vi "merlin.vi"() -> ()   [LabVIEW 2018]
uses:
  classes/Tushars Events Toolkit/Software/Modules/EventClient_ObjectReference.ctl
  Strict Type Controls/Settings Operation.ctl
  <vilib>/Instr/_visa.llb/VISA Configure Serial Port (Instr).vi
  classes/Variable Manager/VariableManager_Bool.vi
  classes/Variable Manager/VariableManager_Double.vi
panel:
  out "Quit":bool
  out "error out":errorcluster
  in  "error in (no error)":errorcluster
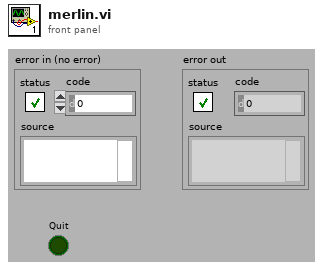
[diagram p1: front panel]
types:
  T1 = typedef "EventClient_ObjectReference.ctl" = refnum<k1>
  T2 = typedef "Settings Operation.ctl" = enum8{"Get Value", "Set Value", "Read File", "Write File", "Write Stored Value"}
  T3 = cluster{"#Stages":enum16{"None", "1 Pole", "2 Pole"}, "Phase":enum16{"1 Phase", "2 Phase"}, "SyncMode":enum16{"Int Chop Off", "Int Chop On", "Ext Chop Off", "Ext Chop On"}, "Time Const":enum16{".003s", ".010s", ".030s", ".100s", ".300s", "1.00s", "3.00s", "10.0s", "30.0s", "100s"}}
  T4 = enum16{"Int Chop Off", "Int Chop On", "Ext Chop Off", "Ext Chop On"}
  T5 = enum16{".003s", ".010s", ".030s", ".100s", ".300s", "1.00s", "3.00s", "10.0s", "30.0s", "100s"}
  T6 = typedef "Settings.ctl" = cluster{"Mono Cr":cluster{"Port":refnum<visa-resource-name>, "baud rate":u32, "data bits":u16, "parity":enum16{"None", "Odd", "Even", "Mark", "Space"}, "stop bits":u16, "flow control":u16, "timeout":u32}, "Merlin":cluster{"Port":refnum<visa-resource-name>, "baud rate":u32, "data bits":u16, "parity":enum16{"None", "Odd", "Even", "Mark", "Space"}, "stop bits":u16, "flow control":u16, "timeout":u32}}
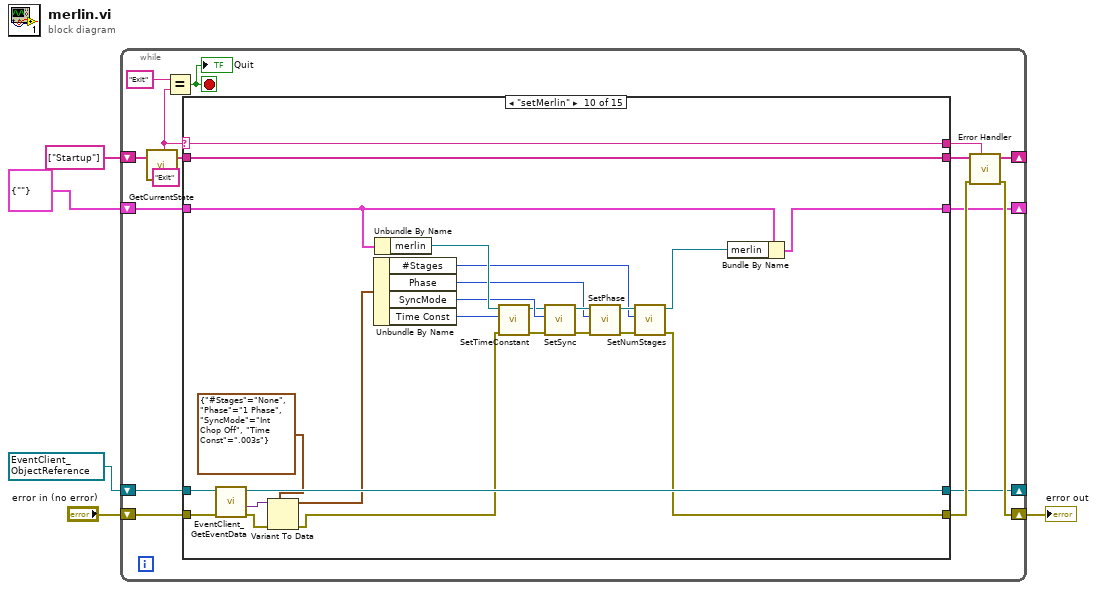
[diagram p0: block diagram]
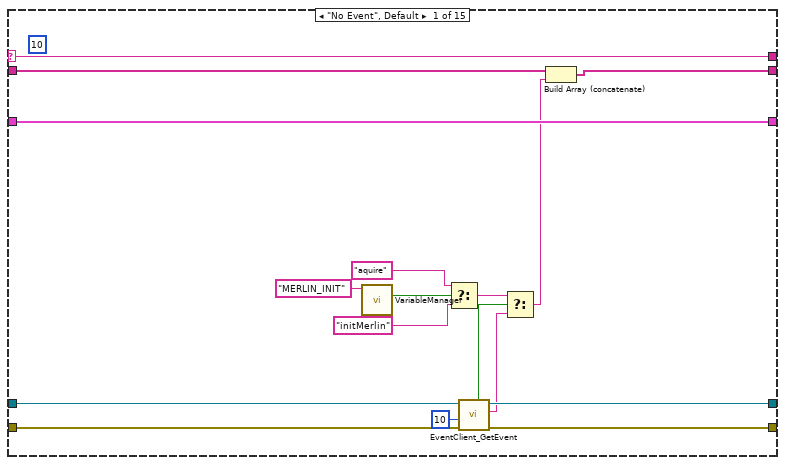
[diagram p2: hidden frame]
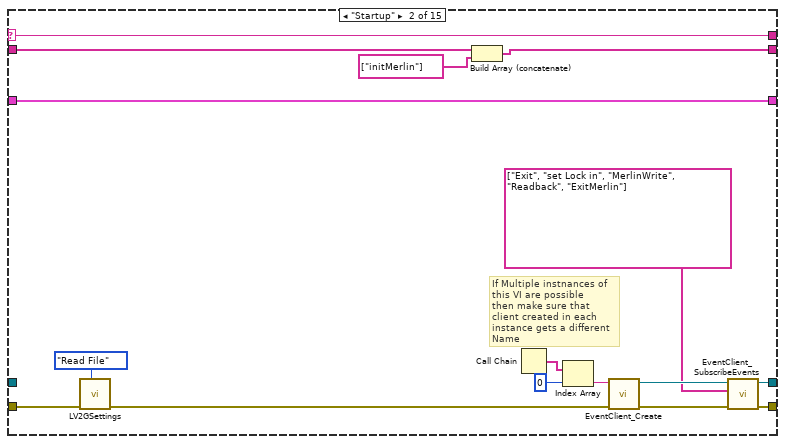
[diagram p3: hidden frame]
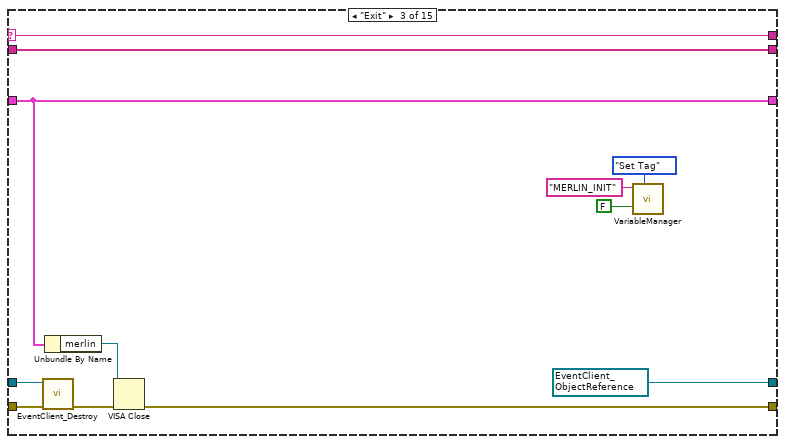
[diagram p4: hidden frame]
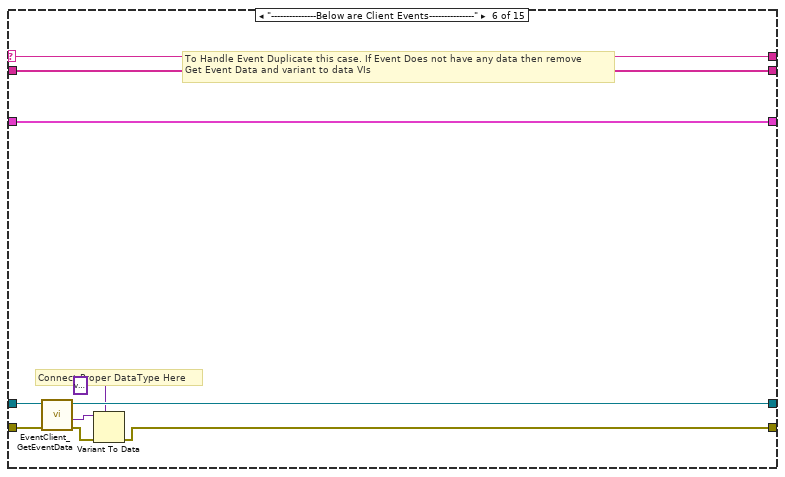
[diagram p7: hidden frame]
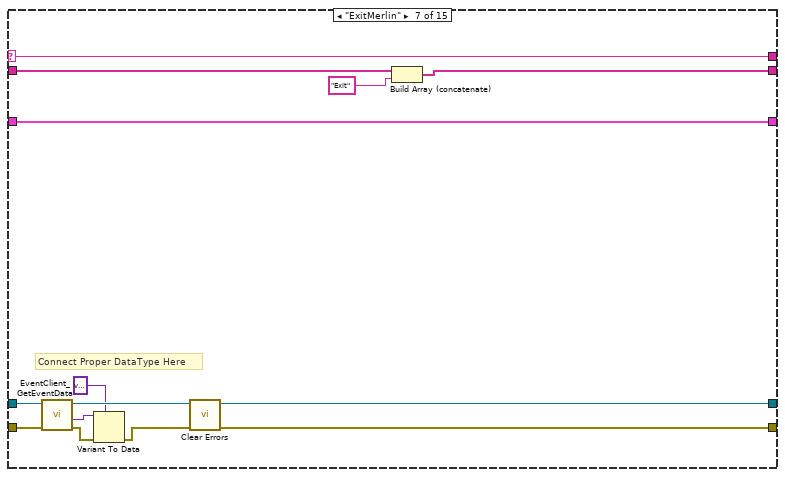
[diagram p8: hidden frame]
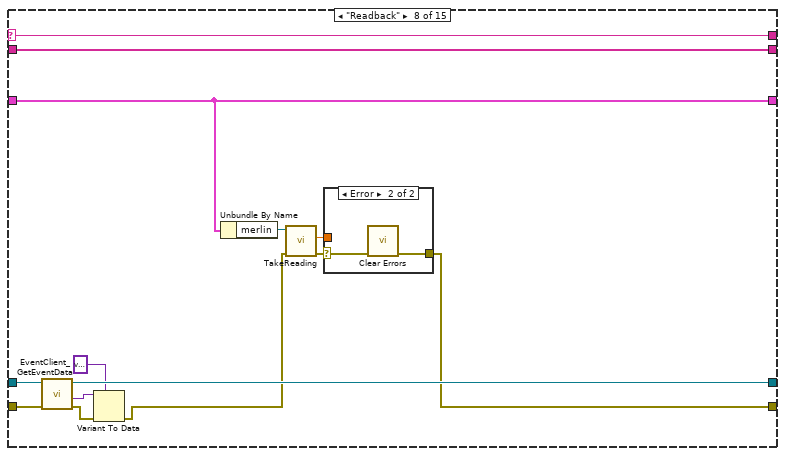
[diagram p9: hidden frame]
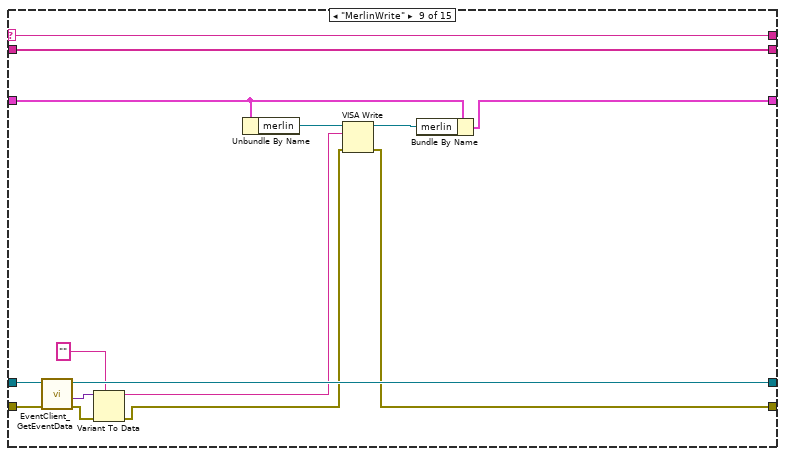
[diagram p11: hidden frame]
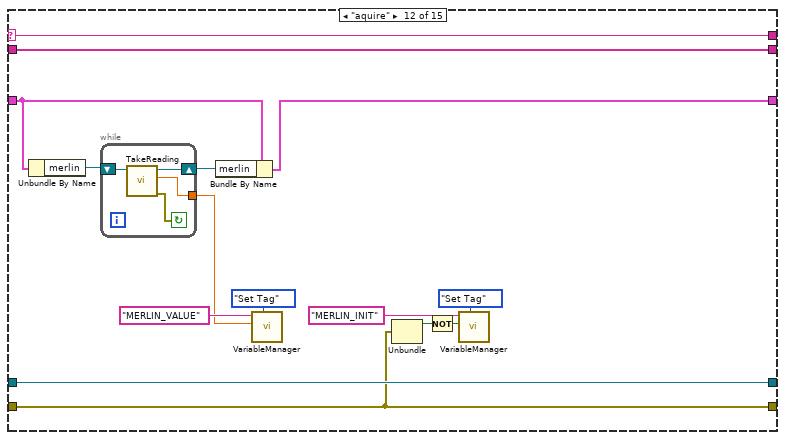
[diagram p13: hidden frame]
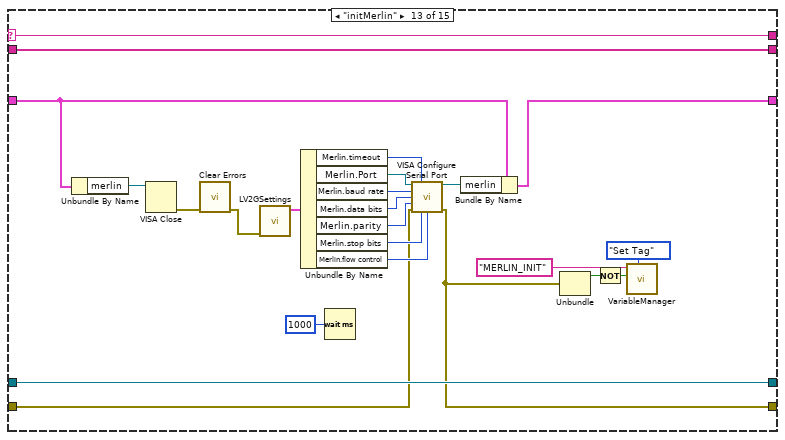
[diagram p14: hidden frame]
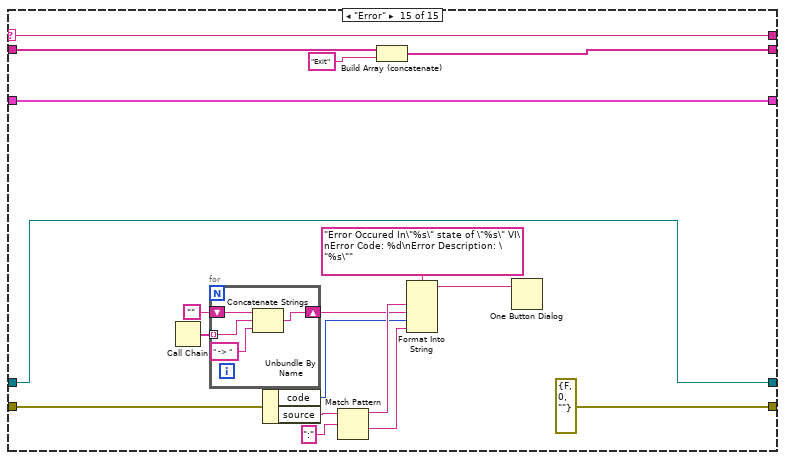
[diagram p16: hidden frame]
diagram:
  w2 = T1 refnum items=["EventClient"] ("reference")
  n1 = while {
    shift-right: [w16] -> _
    shift-left: string[] ["Startup"] ("State Array Out") -> [w20]
    shift-right: [w12] -> w3
    shift-left: "error in (no error)" -> [w13]
    shift-right: [w9] -> _
    shift-left: w2 -> [w8]
    shift-right: [w6] -> _
    shift-left: cluster{"merlin":refnum<visa-resource-name>} {"merlin"=""} -> [w7]
    stop <- w17 stop-if-true
    (unwired) "Exit" ("x")
    n2 = call "GetCurrentState.vi"("State Array In"=w20) -> ("Current State"=w10:string, "State Array Out"=w19:string[])  [unwired: 17 in]
    n3 = Equal?(x="Exit", y=w10) -> (x = y?=w17:bool)
    "Quit" <- w17
    n4 = case shown="\"setMerlin\"" w10 {
      selector: w10 -> [w37 w53 w65 w69 w74 w84 w97 w111 w129 w154 w159 w174 w202 w208 w226]
      tunnel: w19 -> [w29 w52 w64 w70 w75 w85 w98 w112 w130 w155 w160 w175 w203 w207 w213]
      tunnel: [w32 w51 w64 w70 w75 w85 w88 w112 w130 w155 w160 w175 w203 w207 w210] -> w15
      tunnel: [w34 w45 w59 w68 w73 w80 w86 w99 w116 w133 w158 w169 w182 w206 errorcluster {"status"=FALSE, "code"=0, "source"=""} ("error in (no error)")] -> w11
      tunnel: [w37 w53 w65 w69 w74 w84 w97 w111 w129 w154 w159 w174 w202 w208 w226] -> w14
      tunnel: w13 -> [w35 w40 w62 w68 w73 w82 w95 w109 w127 w152 w158 w169 w186 w206 w214]
      tunnel: [w33 w43 w61 w67 w72 w78 w91 w106 w124 w149 w157 w173 w201 w205 w212] -> w9
      tunnel: w8 -> [w36 _ w63 w67 w72 w83 w96 w110 w128 w153 w157 w173 w201 w205 w212]
      tunnel: w7 -> [w30 w41 w58 w66 w71 w76 w89 w101 w121 w145 w156 w166 w189 w204 w211]
      tunnel: [w30 w41 w58 w66 w71 w76 w89 w101 w122 w146 w156 w165 w188 w204 w211] -> w6
      frame "No Event", Default {
        (unwired) 10
        n5 = call-poly "VariableManager.vi"("Tag"="MERLIN_INIT") -> ("Value out"=w27:bool)  [unwired: 7 in, 3 out]
        n6 = Select(t="aquire" ("Tag"), s=w27, f="initMerlin" ("Tag")) -> (s? t:f=w23:string)
        n7 = call "EventClient_GetEvent.vi"("error in (no error)"=w35, "timeout in ms (-1)"=10, "reference"=w36) -> ("error out"=w34:errorcluster, "Name"=w22:string, "reference out"=w33:T1, "timed out?"=w24:bool)  [unwired: 4 in, 1 out]
        n8 = Select(t=w23, s=w24, f=w22) -> (s? t:f=w21:string)
        n9 = Build Array (concatenate)(w29, w21) -> (w32:string[])
      }
      frame "Startup" {
        # "If Multiple instnances of this VI are possible \nthen make sure that client created in each instance gets a different Name"
        n10 = call "LV2GSettings.vi"("Operation"=Settings_Operation."Read File", "error in (no error)"=w40) -> ("error out"=w39:errorcluster)  [unwired: 8 in, 1 out]
        n11 = Build Array (concatenate)(w52, string[] ["initMerlin"] ("State Array Out")) -> (w51:string[])
        n12 = Call Chain() -> (call chain=w49:string[])
        n13 = Index Array(array=w49, index=0) -> (element=w47:string)
        n14 = call "EventClient_Create.vi"("error in (no error)"=w39, "Instance Name"=w47) -> ("error out"=w46:errorcluster, "reference"=w44:T1)  [unwired: 8 in]
        n15 = call "EventClient_SubscribeEvents.vi"("error in (no error)"=w46, "Events"=string[] ["Exit", "set Lock in", "MerlinWrite", "Readback", "ExitMerlin"], "reference"=w44) -> ("error out"=w45:errorcluster, "reference out"=w43:T1)  [unwired: 7 in]
      }
      frame "Exit" {
        w61 = T1 refnum items=["EventClient"] ("reference out")
        n16 = call "EventClient_Destroy.vi"("error in (no error)"=w62, "reference"=w63) -> ("error out"=w60:errorcluster)  [unwired: 9 in]
        n17 = Unbundle By Name(w58) -> ("merlin"=w57:refnum<visa-resource-name>)
        n18 = VISA Close(VISA resource name=w57, error in (no error)=w60) -> (error out=w59:errorcluster)
        n19 = call-poly "VariableManager.vi"("Operation"=enum16{"Get Tag", "Set Tag"}."Set Tag", "Value"=FALSE, "Tag"="MERLIN_INIT") -> ()  [unwired: 5 in, 4 out]
      }
      frame "---------------Below are UI Events---------------" {
        # "This State will never Execute\nIt is added just for improving code readability please do not remove this case"
      }
      frame "---------------Below are Menu Events---------------" {
        # "This State will never Execute\nIt is added just for improving code readability please do not remove this case"
      }
      frame "---------------Below are Client Events---------------" {
        # "To Handle Event Duplicate this case. If Event Does not have any data then remove\nGet Event Data and variant to data VIs"
        # "Connect Proper DataType Here"
        n20 = call "EventClient_GetEventData.vi"("error in (no error)"=w82, "reference"=w83) -> ("error out"=w81:errorcluster, "Data"=w79:variant, "reference out"=w78:T1)  [unwired: 7 in]
        n21 = Variant To Data(error in=w81, type=variant, Variant=w79) -> (error out=w80:errorcluster)  [unwired: 1 out]
      }
      frame "ExitMerlin" {
        # "Connect Proper DataType Here"
        n22 = call "EventClient_GetEventData.vi"("error in (no error)"=w95, "reference"=w96) -> ("error out"=w94:errorcluster, "Data"=w92:variant, "reference out"=w91:T1)  [unwired: 7 in]
        n23 = Variant To Data(error in=w94, type=variant, Variant=w92) -> (error out=w93:errorcluster)  [unwired: 1 out]
        n24 = call <vilib>:"Clear Errors.vi"("error in (no error)"=w93) -> ("error out"=w86:errorcluster)  [unwired: 5 in, 1 out]
        n25 = Build Array (concatenate)(w98, "Exit" ("x")) -> (w88:string[])
      }
      frame "Readback" {
        n26 = call "EventClient_GetEventData.vi"("error in (no error)"=w109, "reference"=w110) -> ("error out"=w108:errorcluster, "Data"=w107:variant, "reference out"=w106:T1)  [unwired: 7 in]
        n27 = Variant To Data(error in=w108, type=variant, Variant=w107) -> (error out=w100:errorcluster)  [unwired: 1 out]
        n28 = Unbundle By Name(w101) -> ("merlin"=w104:refnum<visa-resource-name>)
        n29 = call "TakeReading.vi"("error in"=w100, "Port"=w104) -> ("error out"=w103:errorcluster, "Voltage(mV)"=w102:dbl)  [unwired: 6 in, 2 out]
        n30 = case shown="Error" w103 {
          selector: w103 -> [w113 w115]
          tunnel: w102 -> [_ _]
          tunnel: [w113 w114] -> w99
          frame No Error {
          }
          frame Error {
            n31 = call <vilib>:"Clear Errors.vi"("error in (no error)"=w115) -> ("error out"=w114:errorcluster)  [unwired: 5 in, 1 out]
          }
        }
      }
      frame "MerlinWrite" {
        n32 = call "EventClient_GetEventData.vi"("error in (no error)"=w127, "reference"=w128) -> ("error out"=w126:errorcluster, "Data"=w125:variant, "reference out"=w124:T1)  [unwired: 7 in]
        n33 = Variant To Data(error in=w126, type="", Variant=w125) -> (data=w118:string, error out=w117:errorcluster)
        n34 = Unbundle By Name(w121) -> ("merlin"=w120:refnum<visa-resource-name>)
        n35 = VISA Write(VISA resource name=w120, write buffer=w118, error in (no error)=w117) -> (VISA resource name out=w119:refnum<visa-resource-name>, error out=w116:errorcluster)  [unwired: 1 out]
        n36 = Bundle By Name(cluster=w121, "merlin"=w119) -> (w122:cluster{"merlin":refnum<visa-resource-name>})
      }
      frame "setMerlin" {
        n37 = call "EventClient_GetEventData.vi"("error in (no error)"=w152, "reference"=w153) -> ("error out"=w151:errorcluster, "Data"=w150:variant, "reference out"=w149:T1)  [unwired: 7 in]
        n38 = Variant To Data(error in=w151, type=T3 {"#Stages"=enum."None", "Phase"=enum."1 Phase", "SyncMode"=enum."Int Chop Off", "Time Const"=enum.".003s"}, Variant=w150) -> (data=w147:T3, error out=w134:errorcluster)
        n39 = Unbundle By Name(w147) -> ("#Stages"=w131:enum16{"None", "1 Pole", "2 Pole"}, "Phase"=w132:enum16{"1 Phase", "2 Phase"}, "SyncMode"=w139:T4, "Time Const"=w141:T5)
        n40 = Unbundle By Name(w145) -> ("merlin"=w140:refnum<visa-resource-name>)
        n41 = call "SetTimeConstant.vi"("error in"=w134, "Time Const"=w141, "Port"=w140) -> ("error out"=w144:errorcluster, "Port out"=w138:refnum<visa-resource-name>)  [unwired: 7 in]
        n42 = call "SetSync.vi"("error in"=w144, "SyncMode"=w139, "Port"=w138) -> ("error out"=w143:errorcluster, "Port out"=w137:refnum<visa-resource-name>)  [unwired: 7 in]
        n43 = call "SetPhase.vi"("error in"=w143, "Phase"=w132, "Port"=w137) -> ("error out"=w142:errorcluster, "Port out"=w136:refnum<visa-resource-name>)  [unwired: 7 in]
        n44 = call "SetNumStages.vi"("error in"=w142, "#Stages"=w131, "Port"=w136) -> ("error out"=w133:errorcluster, "Port out"=w135:refnum<visa-resource-name>)  [unwired: 7 in]
        n45 = Bundle By Name(cluster=w145, "merlin"=w135) -> (w146:cluster{"merlin":refnum<visa-resource-name>})
      }
      frame "---------------Below are Subroutine states---------------" {
      }
      frame "aquire" {
        n46 = Unbundle By Name(w166) -> ("merlin"=w167:refnum<visa-resource-name>)
        n47 = while {
          tunnel: [w177] -> w161
          shift-right: [w176] -> w164
          shift-left: w167 -> [w178]
          stop <- w179 continue-if-true
          n48 = call "TakeReading.vi"("Port"=w178) -> ("error out"=w179:errorcluster, "Voltage(mV)"=w177:dbl, "Port out"=w176:refnum<visa-resource-name>)  [unwired: 7 in, 1 out]
        }
        n49 = Bundle By Name(cluster=w166, "merlin"=w164) -> (w165:cluster{"merlin":refnum<visa-resource-name>})
        n50 = call-poly "VariableManager.vi"("Operation"=enum16{"Get Tag", "Set Tag"}."Set Tag", "Value"=w161, "Tag"="MERLIN_VALUE") -> ()  [unwired: 4 in, 5 out]
        n51 = Unbundle(w169) -> ("status"=w171:bool)  [unwired: 2 out]
        n52 = Not(x=w171) -> (.not. x?=w172:bool)
        n53 = call-poly "VariableManager.vi"("Operation"=enum16{"Get Tag", "Set Tag"}."Set Tag", "Value"=w172, "Tag"="MERLIN_INIT") -> ()  [unwired: 5 in, 4 out]
      }
      frame "initMerlin" {
        n54 = Unbundle By Name(w189) -> ("merlin"=w190:refnum<visa-resource-name>)
        n55 = VISA Close(VISA resource name=w190) -> (error out=w192:errorcluster)  [unwired: 1 in]
        n56 = call <vilib>:"Clear Errors.vi"("error in (no error)"=w192) -> ("error out"=w191:errorcluster)  [unwired: 5 in, 1 out]
        n57 = call "LV2GSettings.vi"("error in (no error)"=w191) -> ("Settings out"=w200:T6)  [unwired: 9 in, 1 out]
        n58 = Unbundle By Name(w200) -> ("Merlin.timeout"=w199:u32, "Merlin.Port"=w193:refnum<visa-resource-name>, "Merlin.baud rate"=w198:u32, "Merlin.data bits"=w197:u16, "Merlin.parity"=w196:enum16{"None", "Odd", "Even", "Mark", "Space"}, "Merlin.stop bits"=w195:u16, "Merlin.flow control"=w194:u16)
        n59 = Wait (ms)(milliseconds to wait=u32 1000) -> ()  [unwired: 1 out]
        n60 = call-poly "VISA Configure Serial Port"("VISA resource name"=w193, "timeout (10sec)"=w199, "baud rate (9600)"=w198, "data bits (8)"=w197, "parity (0:none)"=w196, "error in (no error)"=w186, "stop bits (10: 1 bit)"=w195, "flow control (0:none)"=w194) -> ("VISA resource name out"=w187:refnum<visa-resource-name>, "error out"=w182:errorcluster)  [unwired: 6 in]
        n61 = Bundle By Name(cluster=w189, "merlin"=w187) -> (w188:cluster{"merlin":refnum<visa-resource-name>})
        n62 = Unbundle(w182) -> ("status"=w184:bool)  [unwired: 2 out]
        n63 = Not(x=w184) -> (.not. x?=w185:bool)
        n64 = call-poly "VariableManager.vi"("Operation"=enum16{"Get Tag", "Set Tag"}."Set Tag", "Value"=w185, "Tag"="MERLIN_INIT") -> ()  [unwired: 5 in, 4 out]
      }
      frame "---------------Below are Error Handling VIs---------------" {
      }
      frame "Error" {
        n65 = Call Chain() -> (call chain=w221:string[])
        n66 = for {
          tunnel: w221 -> [w229] mode=indexing
          shift-right: [w227] -> w218
          shift-left: "" -> [w230]
          n67 = Concatenate Strings(w230, w229, " -> ") -> (w227:string)
        }
        n68 = Unbundle By Name(w214) -> ("code"=w216:i32, "source"=w215:string)
        n69 = Match Pattern(string=w215, regular expression=":") -> (before substring=w219:string, after substring=w223:string)  [unwired: 1 in, 2 out]
        n70 = Build Array (concatenate)(w213, "Exit" ("x")) -> (w210:string[])
        n71 = Format Into String(format string="Error Occured In\"%s\" state of \"%s\" VI\nError Code: %d\nError Description: \"%s\"", w219, w218, w216, w223) -> (resulting string=w222:string)  [unwired: 2 in, 1 out]
        n72 = One Button Dialog(message=w222) -> ()  [unwired: 1 in, 1 out]
      }
    }
    n73 = call "Error Handler.vi"("Current State"=w14, "error in (no error)"=w11, "Msg Queue In"=w15) -> ("error out"=w12:errorcluster, "Msg Queue Out"=w16:string[])  [unwired: 7 in]
  }
  "error out" <- w3
